vi "Build Insert Statement.vi"(8 "error in (no error)":errorcluster, 9 "TableType":T1, 10 "TableName":string, 11 "KDBConnection in":refnum<class "DBC.lvclass">) -> (0 "error out":errorcluster, 1 "Insert Statement Suffix":string, 2 "Initial Insert Statement Prefix":string, 3 "KDBConnection out":refnum<class "DBC.lvclass">)   [LabVIEW 2020, in "ORM_DBC_Kdb.lvlib" / "DBC.lvclass"]
uses:
  DBC.lvclass
  kdb_TableType_enum.ctl
  DBC.lvclass/DBC.ctl
  <vilib>/Utility/file.llb/Is Path and Not Empty.vi
  <vilib>/Utility/error.llb/Trim Whitespace.vi
  <vilib>/Utility/error.llb/Error Cluster From Error Code.vi
  <vilib>/ErrorRing/Error Ring.xnode
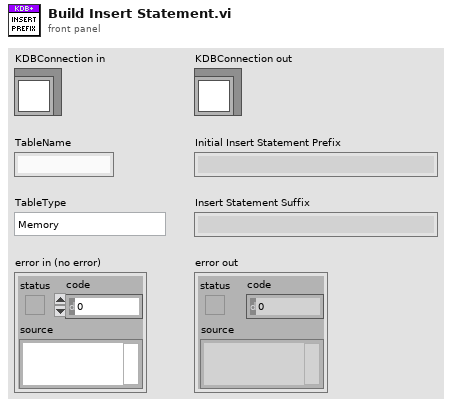
[diagram p1: front panel]
types:
  T1 = typedef "ORM_DBC_Kdb.lvlib/DBC.lvclass/kdb_TableType_enum.ctl" = enum16{"Memory", "Disk_Serialized", "Disk_Splayed", "Disk_Partitioned", "Other"}
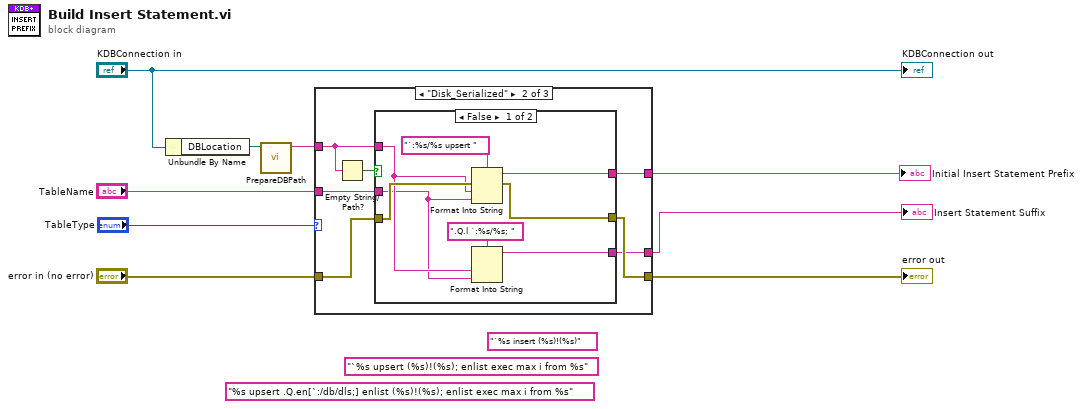
[diagram p0: block diagram]
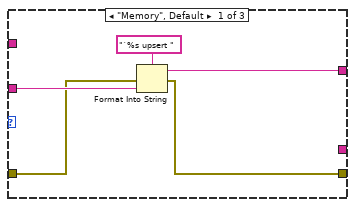
[diagram p2: hidden frame]
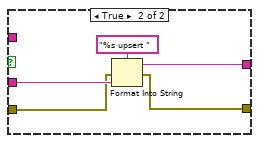
[diagram p3: hidden frame]
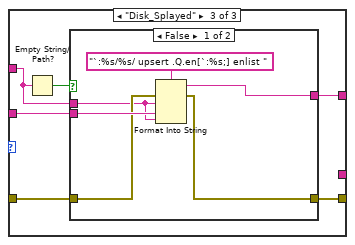
[diagram p4: hidden frame]
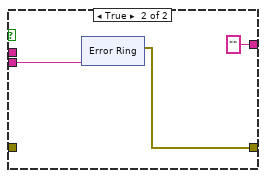
[diagram p5: hidden frame]
diagram:
  (unwired) "%s upsert .Q.en[`:/db/dls;] enlist (%s)!(%s); enlist exec max i from %s"
  (unwired) "`%s insert (%s)!(%s)"
  (unwired) "`%s upsert (%s)!(%s); enlist exec max i from %s"
  n1 = Unbundle By Name("KDBConnection in") -> ("DBLocation"=w8:path)
  n2 = call "PrepareDBPath.vi"("DBLocation"=w8) -> ("result string"=w5:string)  [unwired: 10 in]
  n3 = case shown="\"Disk_Serialized\"" "TableType" {
    tunnel: "TableName" -> [w14 w20 w40]
    tunnel: w5 -> [_ w19 w36]
    tunnel: [w12 w21 w39] -> w4
    tunnel: "error in (no error)" -> [w11 w17 w38]
    tunnel: [w10 w16 w37] -> w2
    tunnel: [_ w15 _] -> w1
    frame "Memory", Default {
      n4 = Format Into String(format string="`%s upsert ", error in=w11, w14) -> (resulting string=w12:string, error out=w10:errorcluster)  [unwired: 1 in]
    }
    frame "Disk_Serialized" {
      n5 = Empty String/Path?(string/path=w19) -> (empty?=w18:bool)
      n6 = case shown="False" w18 {
        tunnel: [w28 w32] -> w21
        tunnel: w20 -> [w22 w33]
        tunnel: w19 -> [w23 _]
        tunnel: w17 -> [w27 w31]
        tunnel: [w26 w30] -> w16
        tunnel: [w24 _] -> w15
        frame False {
          n7 = Format Into String(format string="`:%s/%s upsert ", error in=w27, w23, w22) -> (resulting string=w28:string, error out=w26:errorcluster)  [unwired: 1 in]
          n8 = Format Into String(format string=".Q.l `:%s/%s; ", w23, w22) -> (resulting string=w24:string)  [unwired: 2 in, 1 out]
        }
        frame True {
          n9 = Format Into String(format string="%s upsert ", error in=w31, w33) -> (resulting string=w32:string, error out=w30:errorcluster)  [unwired: 1 in]
        }
      }
    }
    frame "Disk_Splayed" {
      n10 = Empty String/Path?(string/path=w36) -> (empty?=w35:bool)
      n11 = case shown="False" w35 {
        tunnel: w40 -> [w45 w48]
        tunnel: [w44 ""] -> w39
        tunnel: w38 -> [w43 _]
        tunnel: [w42 w47] -> w37
        tunnel: w36 -> [w41 _]
        frame False {
          n12 = Format Into String(format string="`:%s/%s/ upsert .Q.en[`:%s;] enlist ", error in=w43, w41, w45, w41) -> (resulting string=w44:string, error out=w42:errorcluster)  [unwired: 1 in]
        }
        frame True {
          n13 = xnode "Error Ring"("parameter 0"=w48) -> ("error out"=w47:errorcluster)
        }
      }
    }
  }
  "error out" <- w2
  "Initial Insert Statement Prefix" <- w4
  "Insert Statement Suffix" <- w1
  "KDBConnection out" <- "KDBConnection in"
